vi "meth.GetTable.vi"(0 "class.GLue in":refnum<class "class.GLue.lvclass">, 11 "error in (no error)":errorcluster) -> (4 "class.GLue out":refnum<class "class.GLue.lvclass">, 8 "Table":variant, 15 "error out":errorcluster)   [LabVIEW 2014, in "GLue.lvlib" / "class.GLue.lvclass"]
uses:
  class.GLue.lvclass
  class.GLue.lvclass/class.GLue.ctl
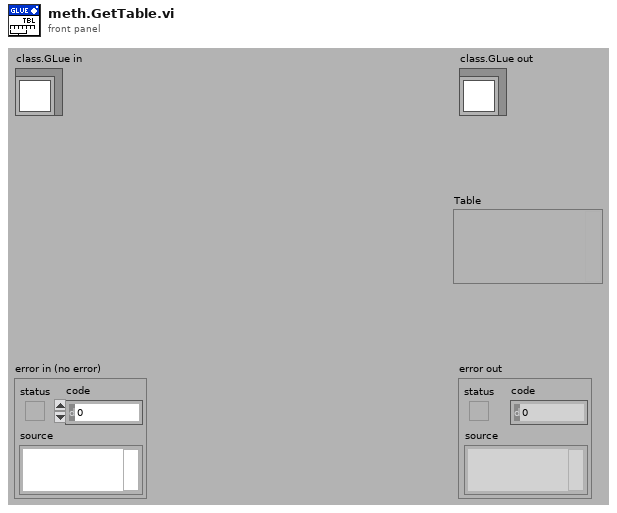
[diagram p1: front panel]
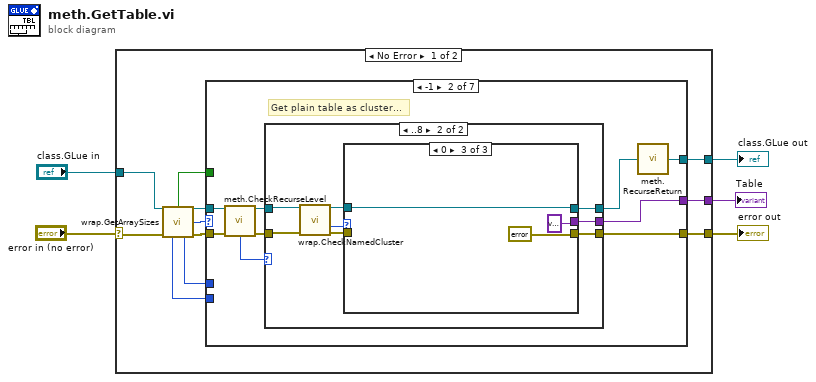
[diagram p0: block diagram]
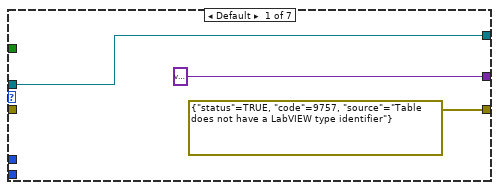
[diagram p2: hidden frame]
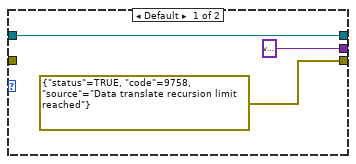
[diagram p3: hidden frame]
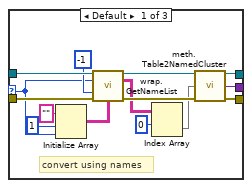
[diagram p4: hidden frame]
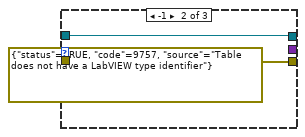
[diagram p5: hidden frame]
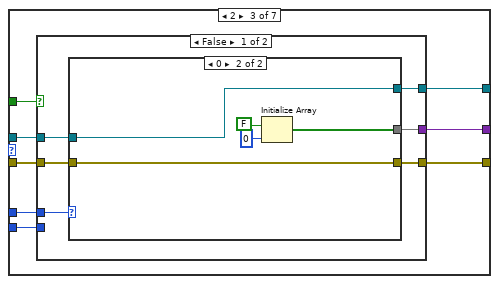
[diagram p6: hidden frame]
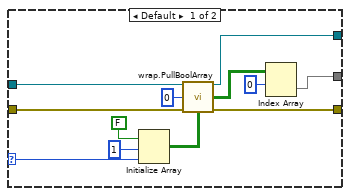
[diagram p7: hidden frame]
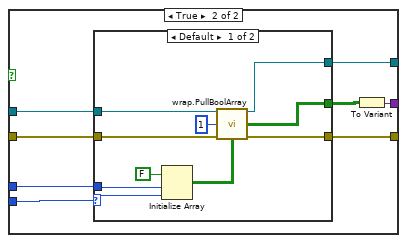
[diagram p8: hidden frame]
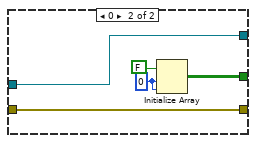
[diagram p9: hidden frame]
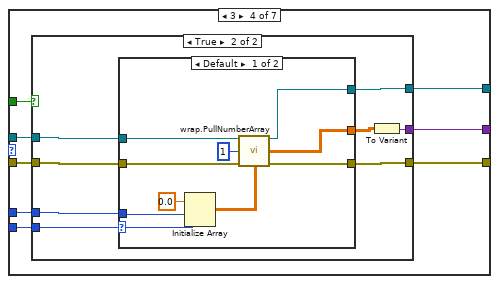
[diagram p10: hidden frame]
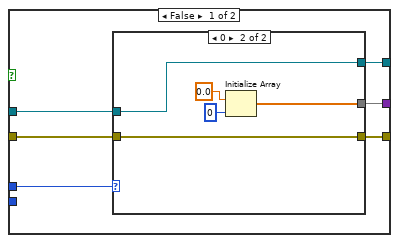
[diagram p11: hidden frame]
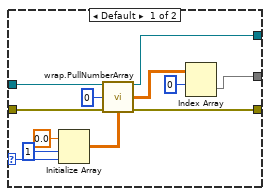
[diagram p12: hidden frame]
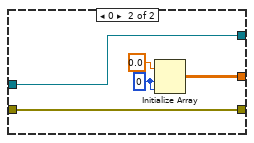
[diagram p13: hidden frame]
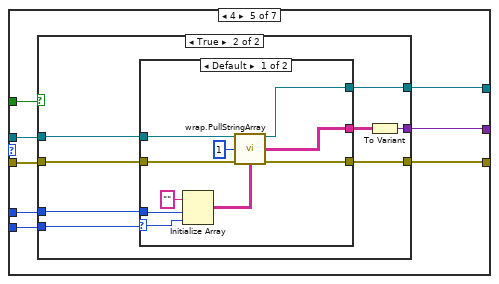
[diagram p14: hidden frame]
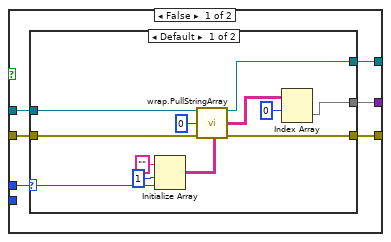
[diagram p15: hidden frame]
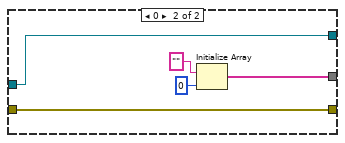
[diagram p16: hidden frame]
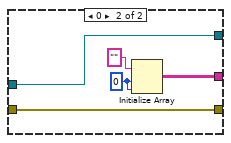
[diagram p17: hidden frame]
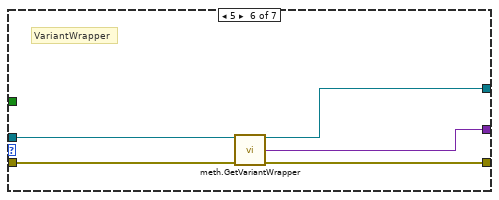
[diagram p18: hidden frame]
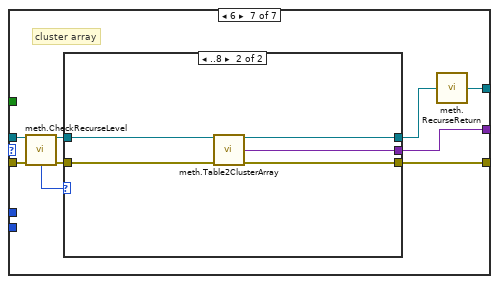
[diagram p19: hidden frame]
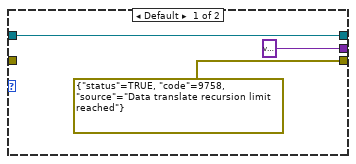
[diagram p20: hidden frame]
diagram:
  n1 = case shown="No Error" "error in (no error)" {
    selector: "error in (no error)" -> [w7 w246]
    tunnel: [w10 w246] -> w4
    tunnel: [w9 w245] -> w2
    tunnel: "class.GLue in" -> [w16 w245]
    tunnel: [w8 variant ("Cluster")] -> w1
    frame No Error {
      n2 = call "wrap.GetArraySizes.vi"("class.GLue in"=w16, "error in (no error)"=w7) -> ("2DArray"=w6:bool, "class.GLue out"=w13:refnum<class "class.GLue.lvclass">, "Array Type"=w15:i32, "Columns"=w11:i32, "Rows"=w12:i32, "error out"=w14:errorcluster)  [unwired: 8 in]
      n3 = case shown="-1" w15 {
        tunnel: w14 -> [_ w25 w62 w119 w168 w224 w231]
        tunnel: w13 -> [w19 w26 w63 w120 w172 w226 w230]
        tunnel: w12 -> [_ _ w61 w118 w170 _ _]
        tunnel: w11 -> [_ _ w60 w117 w169 _ _]
        tunnel: [errorcluster {"status"=TRUE, "code"=9757, "source"="Table does not have a LabVIEW type identifier"} ("error out") w28 w65 w114 w173 w223 w228] -> w10
        tunnel: [w19 w20 w66 w116 w175 w225 w227] -> w9
        tunnel: [variant ("Cluster") w27 w64 w115 w174 w222 w229] -> w8
        tunnel: w6 -> [_ _ w67 w121 w171 _ _]
        frame Default {
        }
        frame -1 {
          # "Get plain table as cluster..."
          n4 = call "meth.CheckRecurseLevel.vi"("class.GLue in"=w26, "error in (no error)"=w25) -> ("class.GLue out"=w23:refnum<class "class.GLue.lvclass">, "Level"=w22:i32, "error out"=w24:errorcluster)  [unwired: 11 in]
          n5 = case shown="..8" w22 {
            tunnel: [errorcluster {"status"=TRUE, "code"=9758, "source"="Data translate recursion limit reached"} ("error out") w39] -> w28
            tunnel: [w31 w37] -> w21
            tunnel: [variant ("Cluster") w38] -> w27
            tunnel: w24 -> [_ w32]
            tunnel: w23 -> [w31 w33]
            frame Default {
            }
            frame ..8 {
              n6 = call "wrap.CheckNamedCluster.vi"("class.GLue in"=w33, "error in (no error)"=w32) -> ("class.GLue out"=w34:refnum<class "class.GLue.lvclass">, "Size"=w36:i32, "error out"=w35:errorcluster)  [unwired: 10 in, 1 out]
              n7 = case shown="0" w36 {
                selector: w36 -> [w49 _ _]
                tunnel: [w46 errorcluster {"status"=TRUE, "code"=9757, "source"="Table does not have a LabVIEW type identifier"} ("error out") errorcluster {"status"=TRUE, "code"=9764, "source"="Empty cluster table cannot be converted into LabVIEW cluster"} ("error out")] -> w39
                tunnel: [w45 _ variant ("Cluster")] -> w38
                tunnel: [w44 w56 w59] -> w37
                tunnel: w35 -> [w52 _ _]
                tunnel: w34 -> [w54 w56 w59]
                frame Default {
                  # "convert using names"
                  n8 = Initialize Array("", 1 ("dimension size"), w49) -> (w48:string[][])
                  n9 = call "wrap.GetNameList.vi"("class.GLue in"=w54, "length"=w49, "index"=-1 ("Index"), "error in (no error)"=w52, "StringArray in"=w48) -> ("class.GLue out"=w43:refnum<class "class.GLue.lvclass">, "StringArray out"=w41:string[][], "error out"=w47:errorcluster)  [unwired: 7 in, 1 out]
                  n10 = Index Array(array=w41, index (row)=0) -> (element=w40:string[])  [unwired: 1 in]
                  n11 = call "meth.Table2NamedCluster.vi"("class.GLue in"=w43, "Names"=w40, "error in"=w47) -> ("class.GLue out"=w44:refnum<class "class.GLue.lvclass">, "Cluster"=w45:variant, "error out"=w46:errorcluster)  [unwired: 10 in]
                }
                frame -1 {
                }
                frame 0 {
                }
              }
            }
          }
          n12 = call "meth.RecurseReturn.vi"("class.GLue in"=w21) -> ("class.GLue out"=w20:refnum<class "class.GLue.lvclass">)  [unwired: 14 in]
        }
        frame 2 {
          n13 = case shown="False" w67 {
            tunnel: w63 -> [w69 w95]
            tunnel: w62 -> [w71 w96]
            tunnel: [w68 w94] -> w66
            tunnel: [w70 w93] -> w65
            tunnel: [w72 w91] -> w64
            tunnel: w61 -> [w73 w97]
            tunnel: w60 -> [_ w98]
            frame False {
              n14 = case shown="0" w73 {
                selector: w73 -> [w75 _]
                tunnel: [w78 w88] -> w72
                tunnel: w71 -> [w84 w87]
                tunnel: [w77 w87] -> w70
                tunnel: w69 -> [w83 w86]
                tunnel: [w81 w86] -> w68
                frame Default {
                  n15 = Initialize Array(FALSE, 1 ("dimension size"), w75) -> (w82:bool[][])
                  n16 = call "wrap.PullBoolArray.vi"("class.GLue in"=w83, "Is2d"=0, "error in (no error)"=w84, "BoolArray in"=w82) -> ("class.GLue out"=w81:refnum<class "class.GLue.lvclass">, "BoolArray out"=w79:bool[][], "error out"=w77:errorcluster)  [unwired: 9 in]
                  n17 = Index Array(array=w79, index (row)=0) -> (element=w78:bool[])  [unwired: 1 in]
                }
                frame 0 {
                  n18 = Initialize Array(FALSE, 0 ("dimension size")) -> (w88:bool[])
                }
              }
            }
            frame True {
              n19 = case shown="Default" w98 {
                selector: w98 -> [w102 _]
                tunnel: w97 -> [w103 _]
                tunnel: [w100 w111] -> w92
                tunnel: w96 -> [w106 w110]
                tunnel: w95 -> [w105 w109]
                tunnel: [w104 w109] -> w94
                tunnel: [w101 w110] -> w93
                frame Default {
                  n20 = Initialize Array(FALSE, w103, w102) -> (w107:bool[][])
                  n21 = call "wrap.PullBoolArray.vi"("class.GLue in"=w105, "Is2d"=1, "error in (no error)"=w106, "BoolArray in"=w107) -> ("class.GLue out"=w104:refnum<class "class.GLue.lvclass">, "BoolArray out"=w100:bool[][], "error out"=w101:errorcluster)  [unwired: 9 in]
                }
                frame 0 {
                  w112 = 0 ("dimension size")
                  n22 = Initialize Array(FALSE, w112, w112) -> (w111:bool[][])
                }
              }
              n23 = To Variant(anything=w92) -> (Variant=w91:variant)
            }
          }
        }
        frame 3 {
          n24 = case shown="True" w121 {
            tunnel: w120 -> [w123 w149]
            tunnel: w119 -> [w125 w150]
            tunnel: [w122 w148] -> w116
            tunnel: [w124 w147] -> w114
            tunnel: [w126 w145] -> w115
            tunnel: w118 -> [w127 w151]
            tunnel: w117 -> [_ w152]
            frame False {
              n25 = case shown="0" w127 {
                selector: w127 -> [w137 _]
                tunnel: [w129 w143] -> w126
                tunnel: w125 -> [w135 w142]
                tunnel: [w131 w142] -> w124
                tunnel: w123 -> [w134 w141]
                tunnel: [w133 w141] -> w122
                frame Default {
                  n26 = Initialize Array(0.0, 1 ("dimension size"), w137) -> (w130:dbl[][])
                  n27 = call "wrap.PullNumberArray.vi"("class.GLue in"=w134, "Is2d"=0, "error in (no error)"=w135, "FloatArray in"=w130) -> ("class.GLue out"=w133:refnum<class "class.GLue.lvclass">, "FloatArray out"=w132:dbl[][], "error out"=w131:errorcluster)  [unwired: 9 in]
                  n28 = Index Array(array=w132, index (row)=0) -> (element=w129:dbl[])  [unwired: 1 in]
                }
                frame 0 {
                  n29 = Initialize Array(0.0 ("dimension size"), 0 ("dimension size")) -> (w143:dbl[])
                }
              }
            }
            frame True {
              n30 = case shown="Default" w152 {
                selector: w152 -> [w161 _]
                tunnel: w151 -> [w162 _]
                tunnel: [w157 w166] -> w146
                tunnel: w150 -> [w159 w165]
                tunnel: w149 -> [w160 w164]
                tunnel: [w156 w164] -> w148
                tunnel: [w155 w165] -> w147
                frame Default {
                  n31 = Initialize Array(0.0 ("dimension size"), w162, w161) -> (w158:dbl[][])
                  n32 = call "wrap.PullNumberArray.vi"("class.GLue in"=w160, "Is2d"=1, "error in (no error)"=w159, "FloatArray in"=w158) -> ("class.GLue out"=w156:refnum<class "class.GLue.lvclass">, "FloatArray out"=w157:dbl[][], "error out"=w155:errorcluster)  [unwired: 9 in]
                }
                frame 0 {
                  w167 = 0 ("dimension size")
                  n33 = Initialize Array(0.0 ("dimension size"), w167, w167) -> (w166:dbl[][])
                }
              }
              n34 = To Variant(anything=w146) -> (Variant=w145:variant)
            }
          }
        }
        frame 4 {
          n35 = case shown="True" w171 {
            tunnel: w172 -> [w177 w203]
            tunnel: w168 -> [w179 w204]
            tunnel: [w176 w202] -> w175
            tunnel: [w178 w201] -> w173
            tunnel: [w180 w199] -> w174
            tunnel: w170 -> [w181 w205]
            tunnel: w169 -> [_ w206]
            frame False {
              n36 = case shown="Default" w181 {
                selector: w181 -> [w191 _]
                tunnel: [w190 w197] -> w180
                tunnel: w179 -> [w186 w196]
                tunnel: [w185 w196] -> w178
                tunnel: w177 -> [w188 w195]
                tunnel: [w187 w195] -> w176
                frame Default {
                  n37 = Initialize Array("", 1 ("dimension size"), w191) -> (w184:string[][])
                  n38 = call "wrap.PullStringArray.vi"("class.GLue in"=w188, "Is2d"=0, "error in (no error)"=w186, "StringArray in"=w184) -> ("class.GLue out"=w187:refnum<class "class.GLue.lvclass">, "StringArray out"=w183:string[][], "error out"=w185:errorcluster)  [unwired: 9 in]
                  n39 = Index Array(array=w183, index (row)=0) -> (element=w190:string[])  [unwired: 1 in]
                }
                frame 0 {
                  n40 = Initialize Array("", 0 ("dimension size")) -> (w197:string[])
                }
              }
            }
            frame True {
              n41 = case shown="Default" w206 {
                selector: w206 -> [w215 _]
                tunnel: w205 -> [w216 _]
                tunnel: [w209 w220] -> w200
                tunnel: w204 -> [w212 w219]
                tunnel: w203 -> [w214 w218]
                tunnel: [w213 w218] -> w202
                tunnel: [w211 w219] -> w201
                frame Default {
                  n42 = Initialize Array("", w216, w215) -> (w210:string[][])
                  n43 = call "wrap.PullStringArray.vi"("class.GLue in"=w214, "Is2d"=1, "error in (no error)"=w212, "StringArray in"=w210) -> ("class.GLue out"=w213:refnum<class "class.GLue.lvclass">, "StringArray out"=w209:string[][], "error out"=w211:errorcluster)  [unwired: 9 in]
                }
                frame 0 {
                  w221 = 0 ("dimension size")
                  n44 = Initialize Array("", w221, w221) -> (w220:string[][])
                }
              }
              n45 = To Variant(anything=w200) -> (Variant=w199:variant)
            }
          }
        }
        frame 5 {
          # "VariantWrapper"
          n46 = call "meth.GetVariantWrapper.vi"("class.GLue in"=w226, "error in"=w224) -> ("class.GLue out"=w225:refnum<class "class.GLue.lvclass">, "Variant"=w222:variant, "error out"=w223:errorcluster)  [unwired: 11 in]
        }
        frame 6 {
          # "cluster array"
          n47 = call "meth.CheckRecurseLevel.vi"("class.GLue in"=w230, "error in (no error)"=w231) -> ("class.GLue out"=w234:refnum<class "class.GLue.lvclass">, "Level"=w233:i32, "error out"=w235:errorcluster)  [unwired: 11 in]
          n48 = case shown="..8" w233 {
            tunnel: [errorcluster {"status"=TRUE, "code"=9758, "source"="Data translate recursion limit reached"} ("error out") w240] -> w228
            tunnel: [w238 w241] -> w232
            tunnel: [variant ("Cluster") w239] -> w229
            tunnel: w235 -> [_ w242]
            tunnel: w234 -> [w238 w243]
            frame Default {
            }
            frame ..8 {
              n49 = call "meth.Table2ClusterArray.vi"("class.GLue in"=w243, "error in"=w242) -> ("class.GLue out"=w241:refnum<class "class.GLue.lvclass">, "Cluster"=w239:variant, "error out"=w240:errorcluster)  [unwired: 11 in]
            }
          }
          n50 = call "meth.RecurseReturn.vi"("class.GLue in"=w232) -> ("class.GLue out"=w227:refnum<class "class.GLue.lvclass">)  [unwired: 14 in]
        }
      }
    }
    frame Error {
    }
  }
  "error out" <- w4
  "class.GLue out" <- w2
  "Table" <- w1
